vi "stepper graphics controller -- V3.vi"(6 "stepper motor state":T2, 7 "slider setter action":T3, 8 "stepper graphics internal state":T1, 10 "value":dbl=1.0 format="%#_13g") -> (0 "stepper graphics internal state OUT":T1)   [LabVIEW 2018]
uses:
  slider setter action.ctl
  stepper motor state.ctl
  stepper graphics internal state.ctl
  2Dwindow.ctl
  slider action.ctl
  cursor action.ctl
  generate linear region.vi
  generate linear region --complex -- win cen.vi
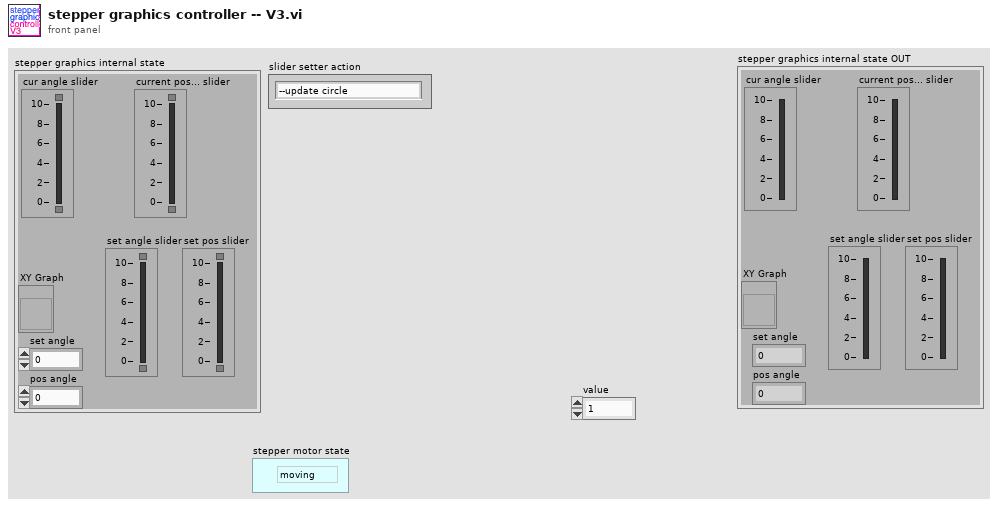
[diagram p1: front panel]
types:
  T1 = typedef "stepper graphics internal state.ctl" = cluster{"set pos slider":refnum<vi>, "cur angle slider":refnum<vi>, "XY Graph":refnum<vi>, "set angle":dbl, "pos angle":dbl, "set angle slider":refnum<vi>, "current pos... slider":refnum<vi>}
  T2 = typedef "stepper motor state.ctl" = enum16{"moving", "stopped"}
  T3 = typedef "slider setter action.ctl" = enum16{"--update circle", "set step slider moves", "cursor moves", "current pos changed", "init", "void", "--draw current lie", "--draw set line", "--move current step slider", "--move set step slider", "--draw limit lines", "check", "--move set angle slider", "--move current angle slider", "set angle slider moves", "--move cursor", "set set step", "set current step"}
  T4 = typedef "2Dwindow.ctl" = cluster{"window y":dbl, "center x":dbl, "center y":dbl, "window x":dbl}
  T5 = typedef "slider action.ctl" = enum16{"check", "copy range", "set from value", "set from ratio", "set from slider", "read using other slider"}
  T6 = typedef "cursor action.ctl" = enum16{"range", "read", "write", "check", "zoom out", "smart zoom out", "zoom to aspect ratio 1", "zoom to win", "zoom out 20%", "zoom in 20%", "-empty", "smart zoom out&aspect", "move range left 20%", "move range right 20%", "move range up 20%", "move range down 20%", "zoom to X win", "zoom to Y win", "zoom out X", "zoom out Y", "zoom in X", "zoom in Y", "check plot scale"}
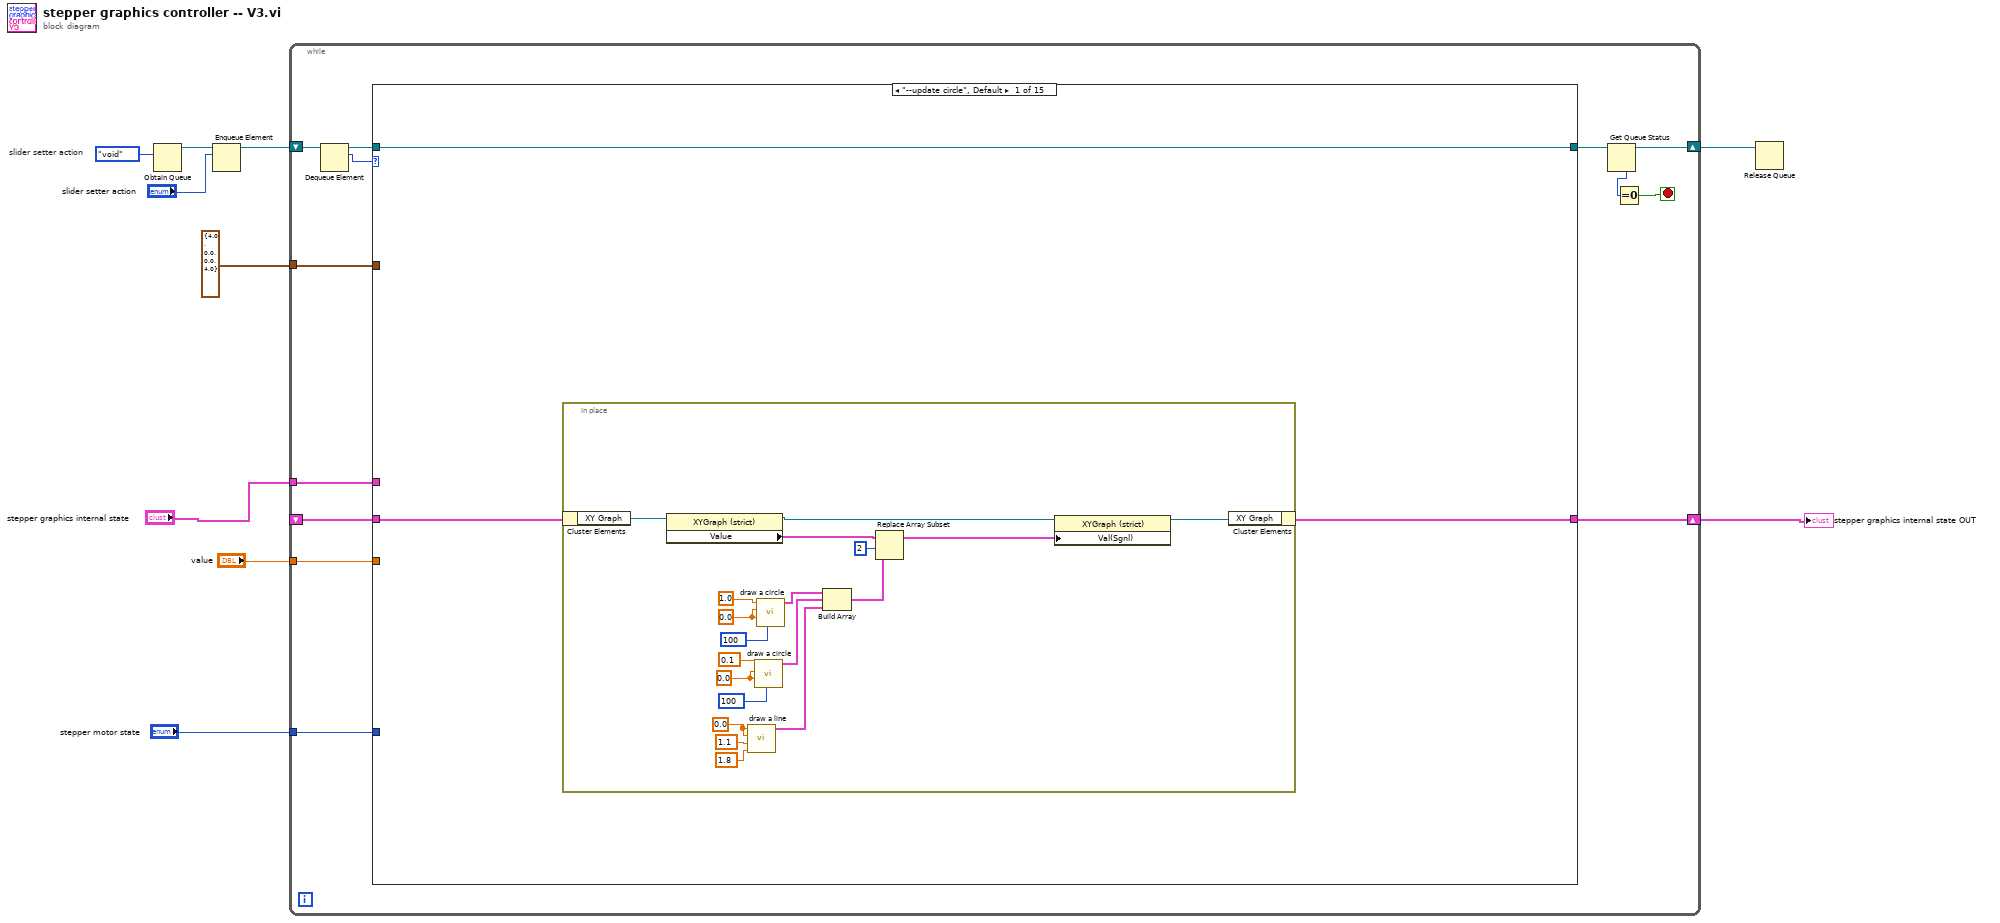
[diagram p0: block diagram]
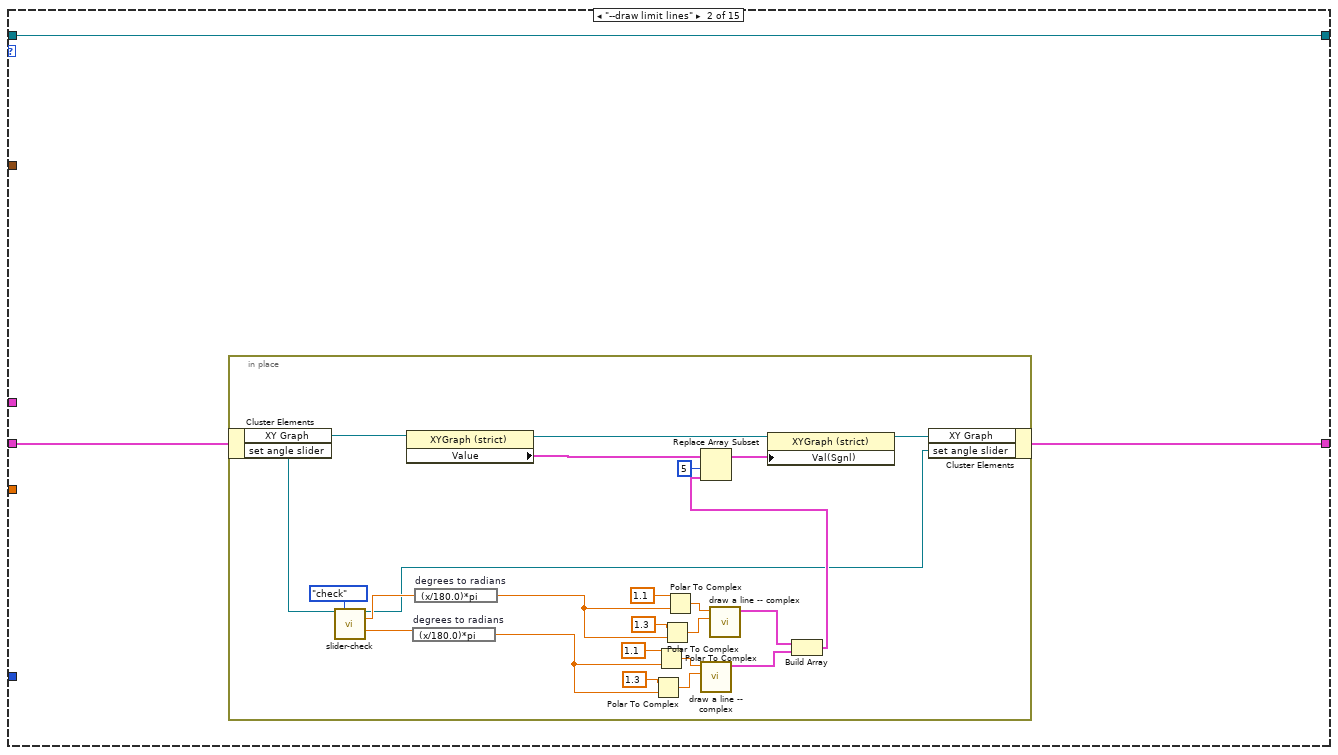
[diagram p2: hidden frame]
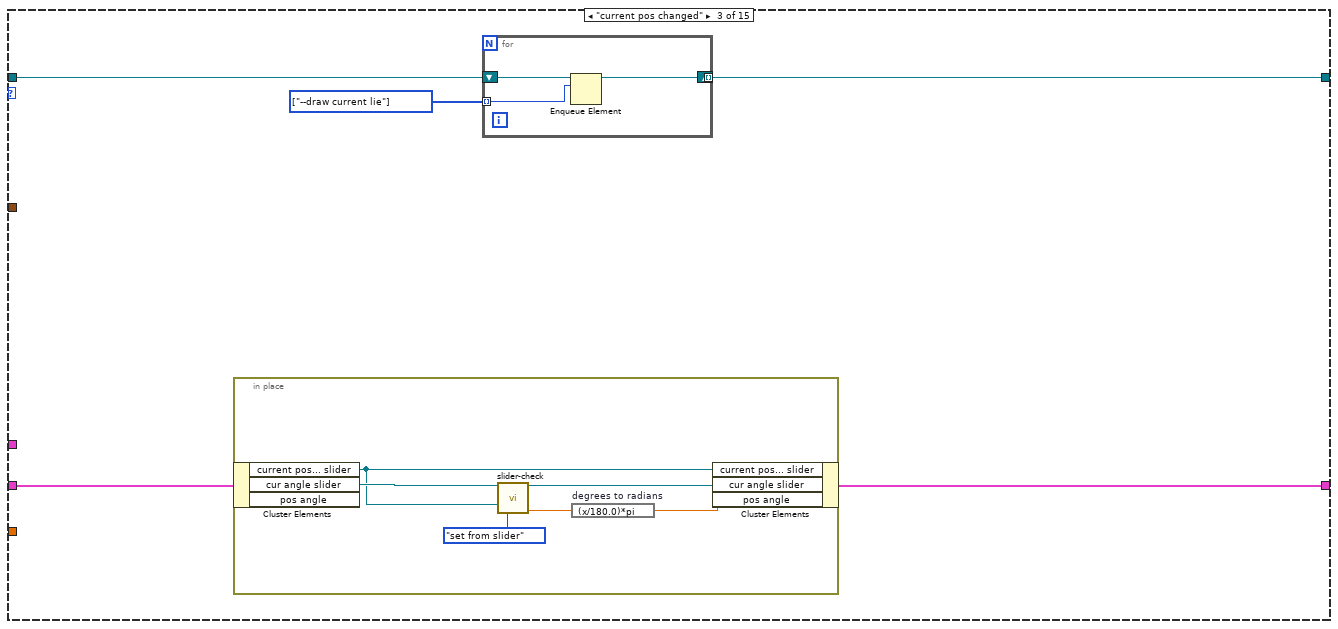
[diagram p3: hidden frame]
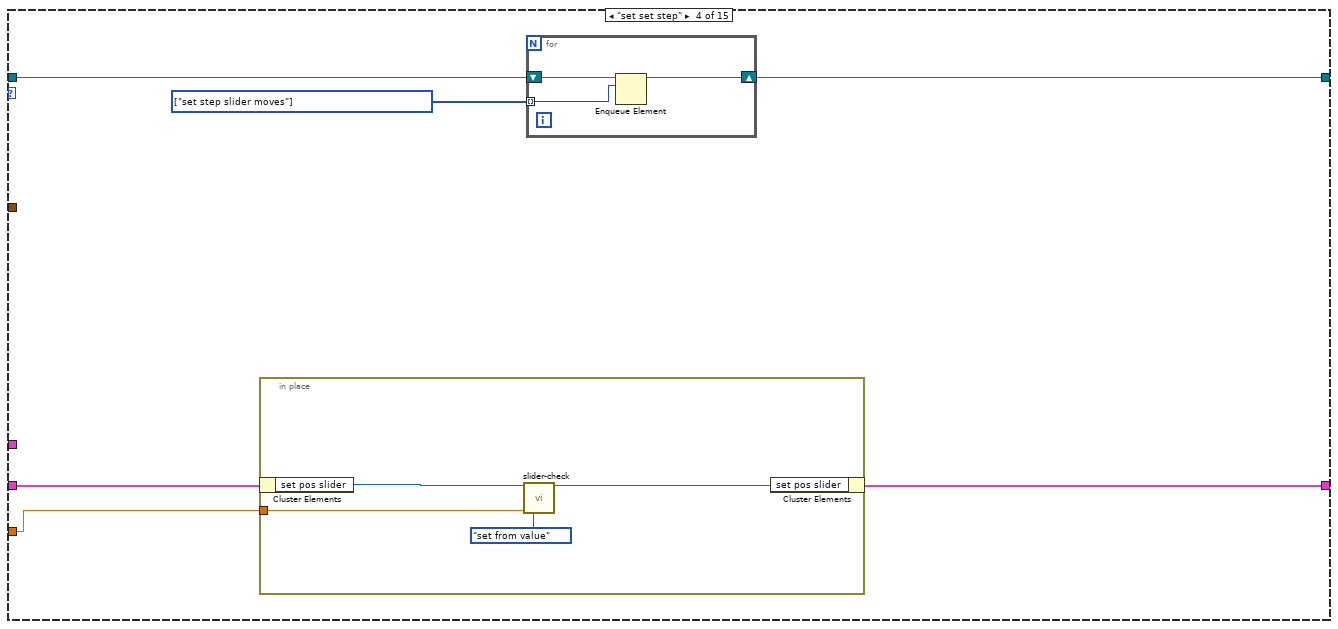
[diagram p4: hidden frame]
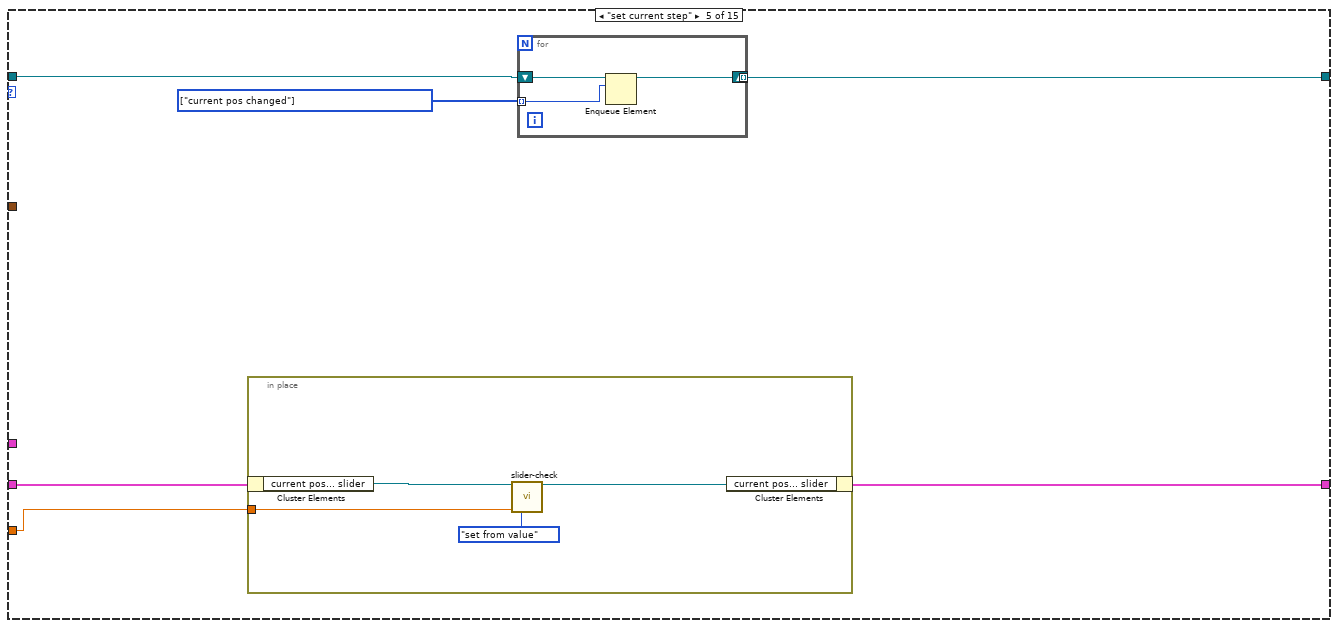
[diagram p5: hidden frame]
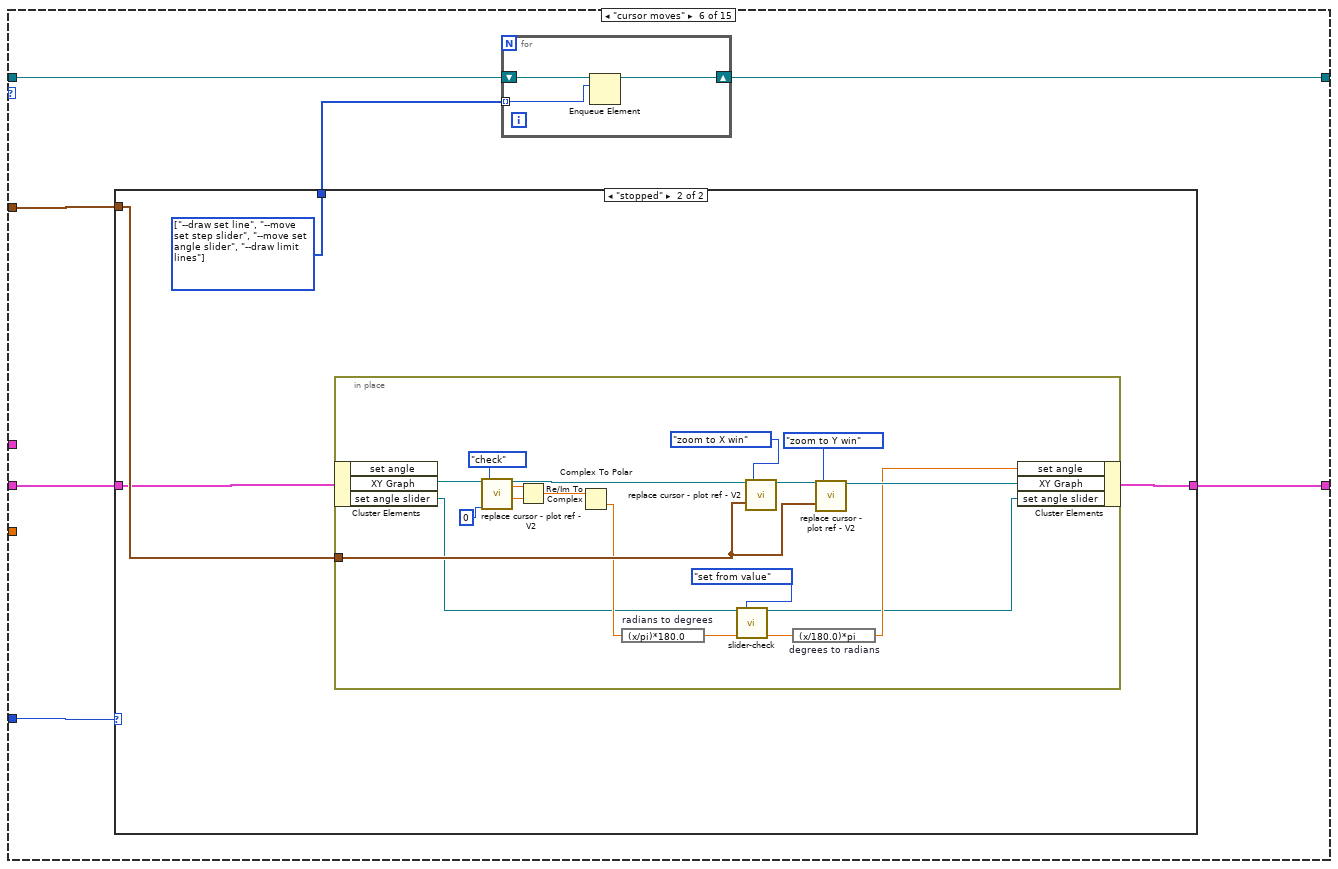
[diagram p6: hidden frame]
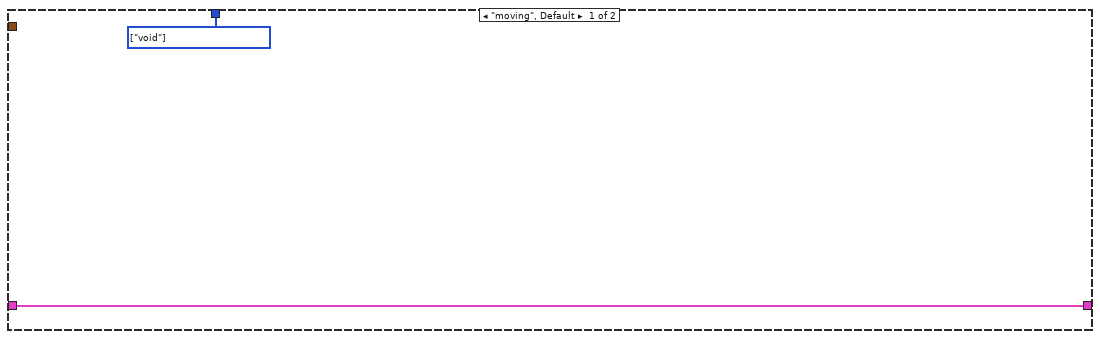
[diagram p7: hidden frame]
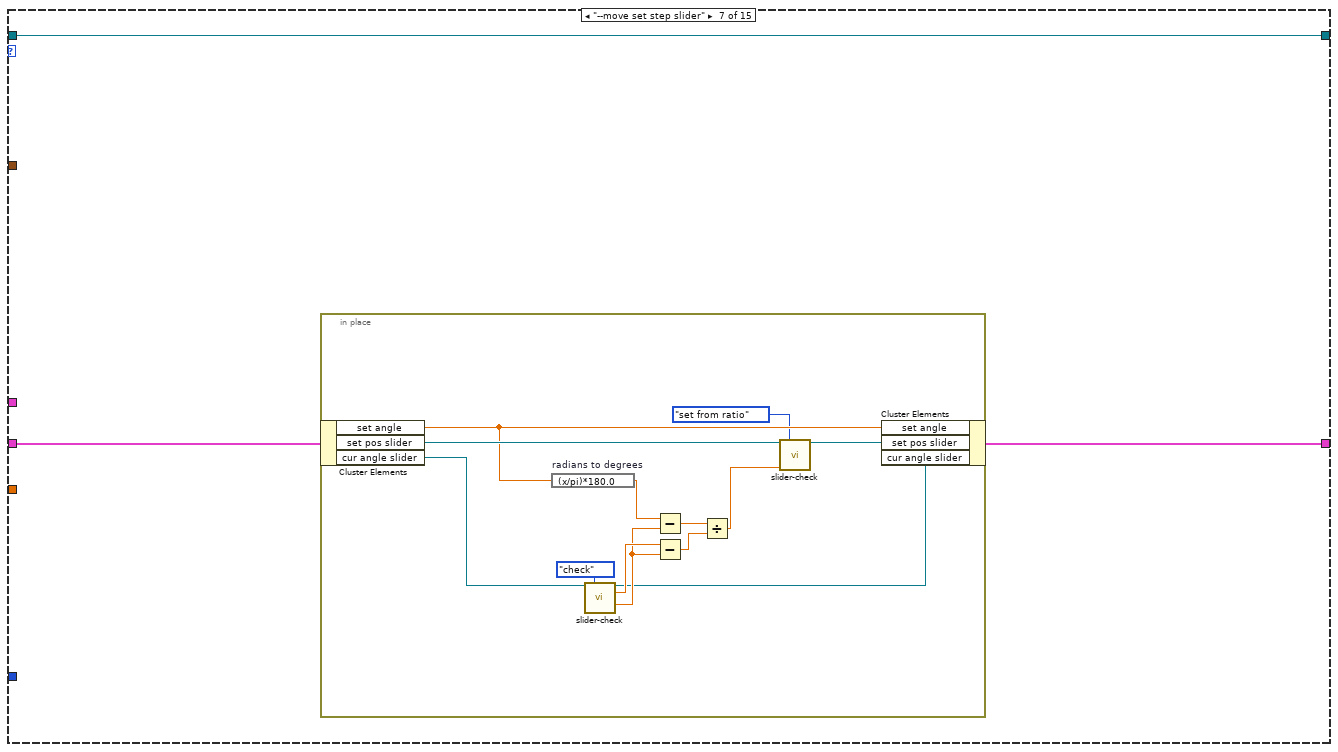
[diagram p8: hidden frame]
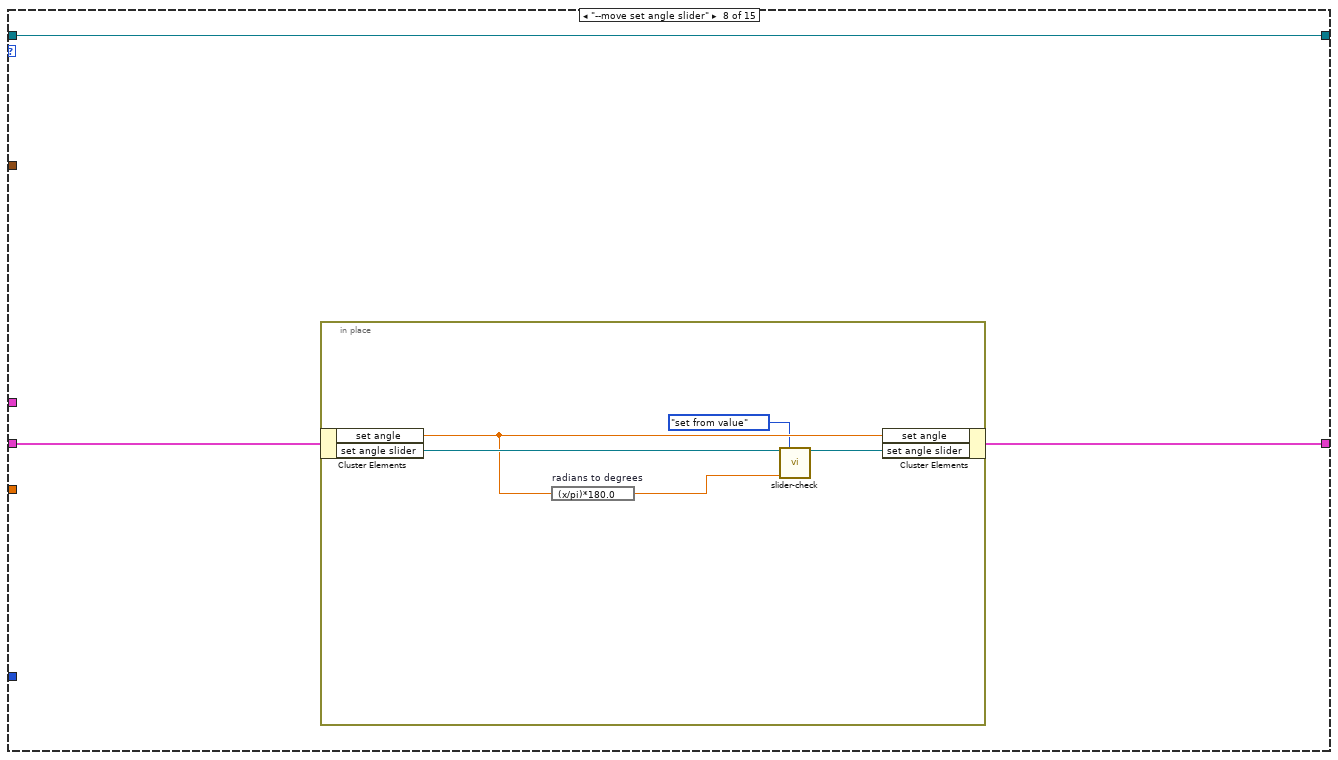
[diagram p9: hidden frame]
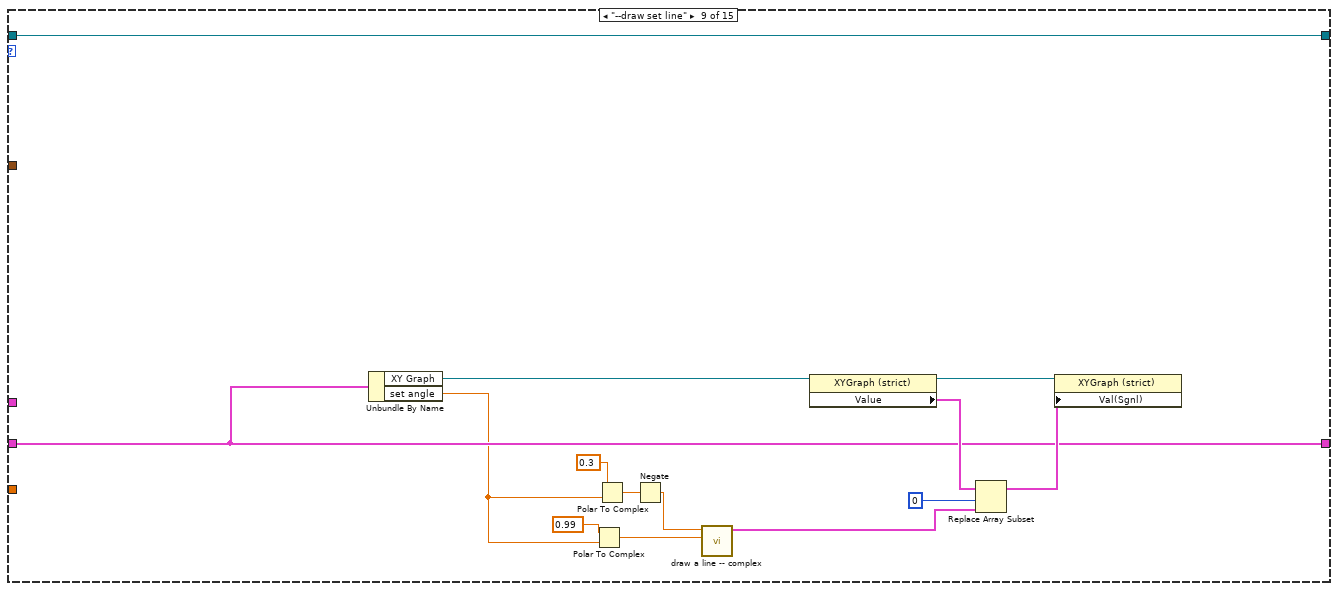
[diagram p10: hidden frame]
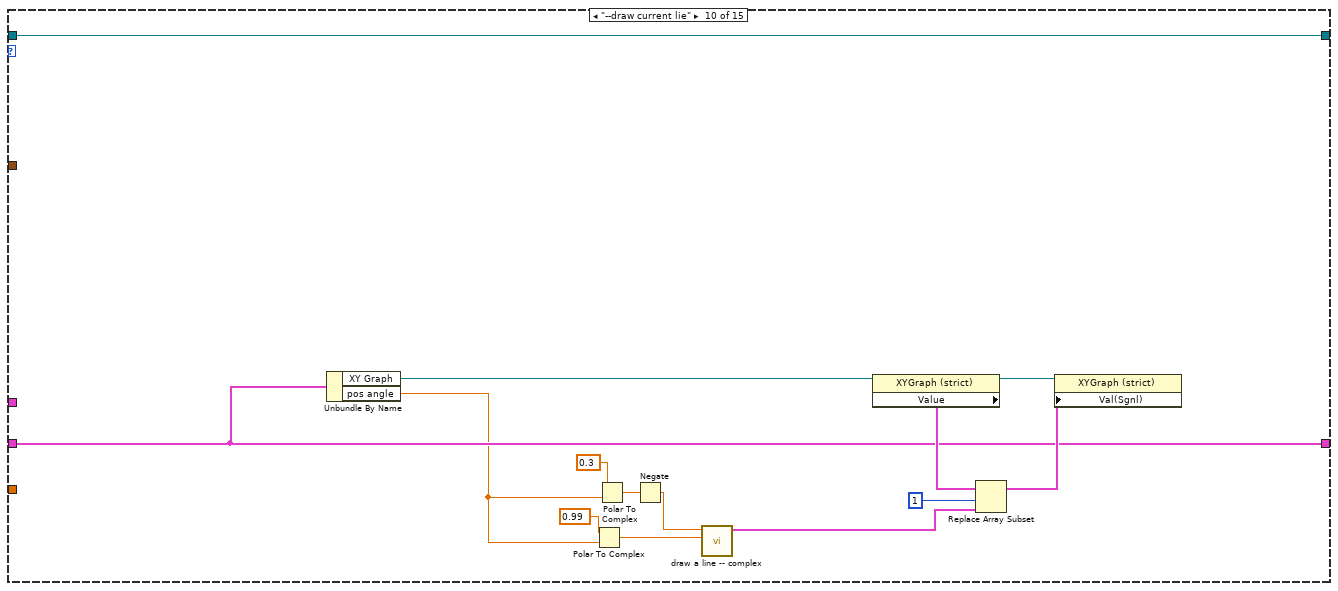
[diagram p11: hidden frame]
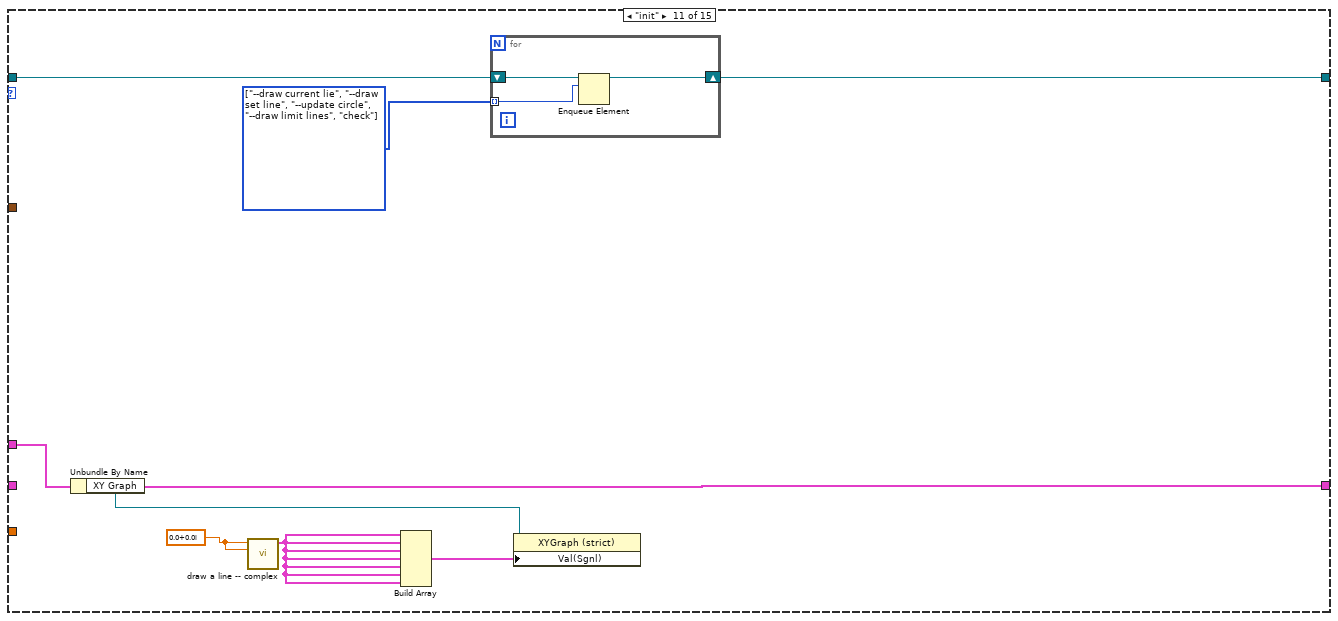
[diagram p12: hidden frame]
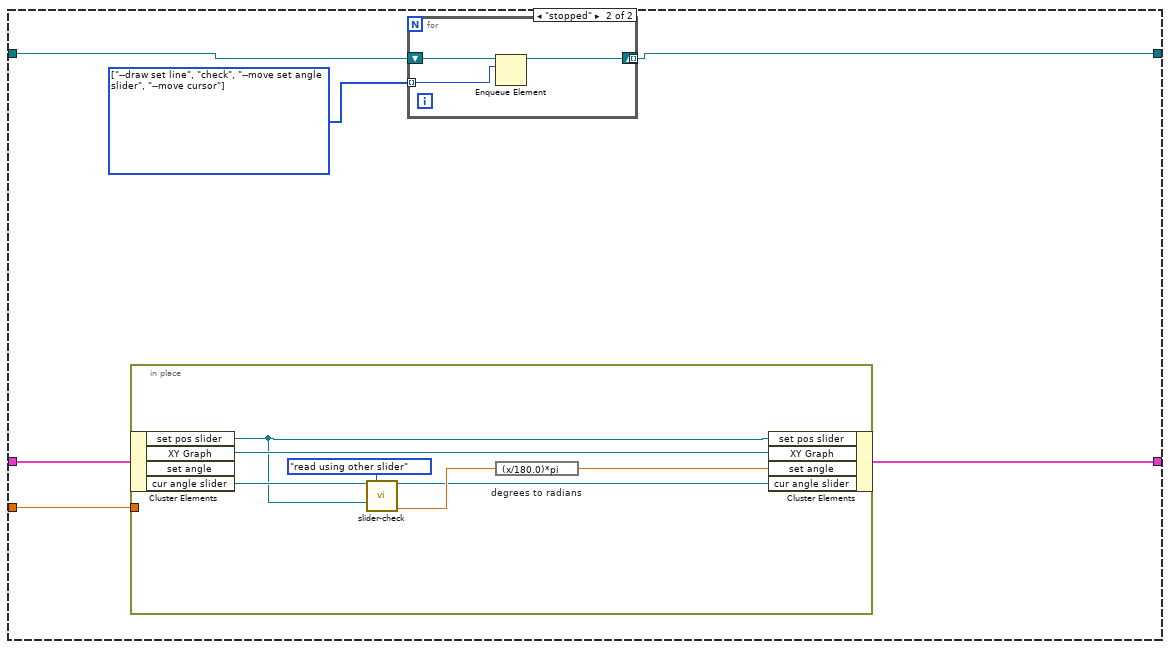
[diagram p14: hidden frame]
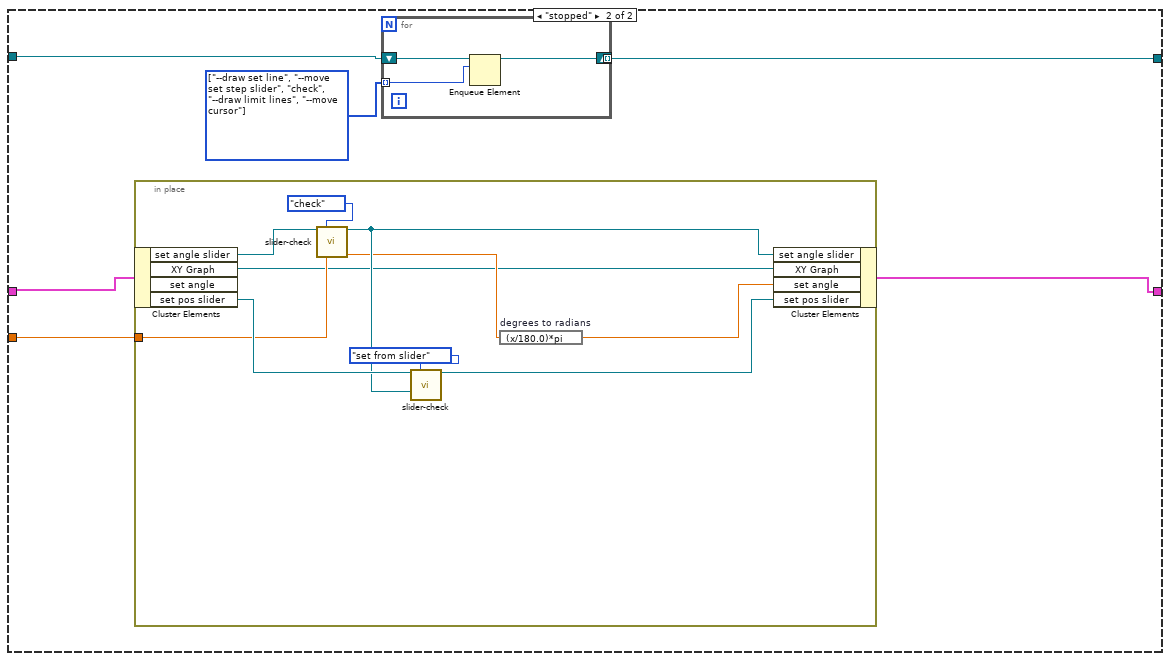
[diagram p16: hidden frame]
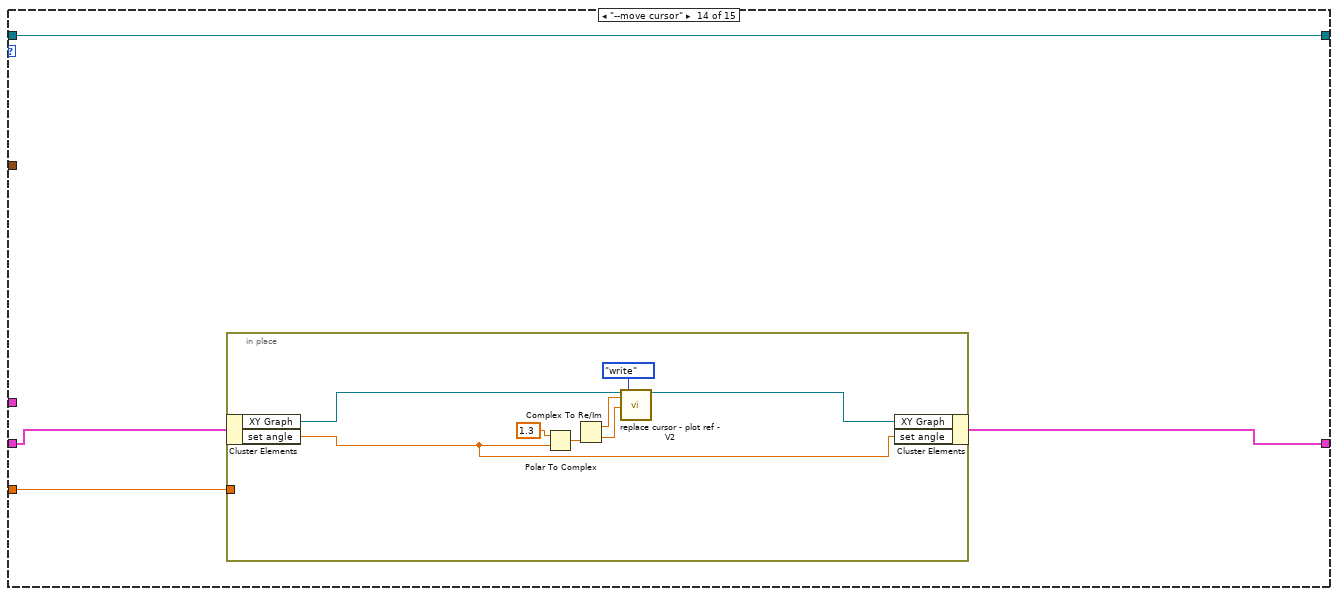
[diagram p17: hidden frame]
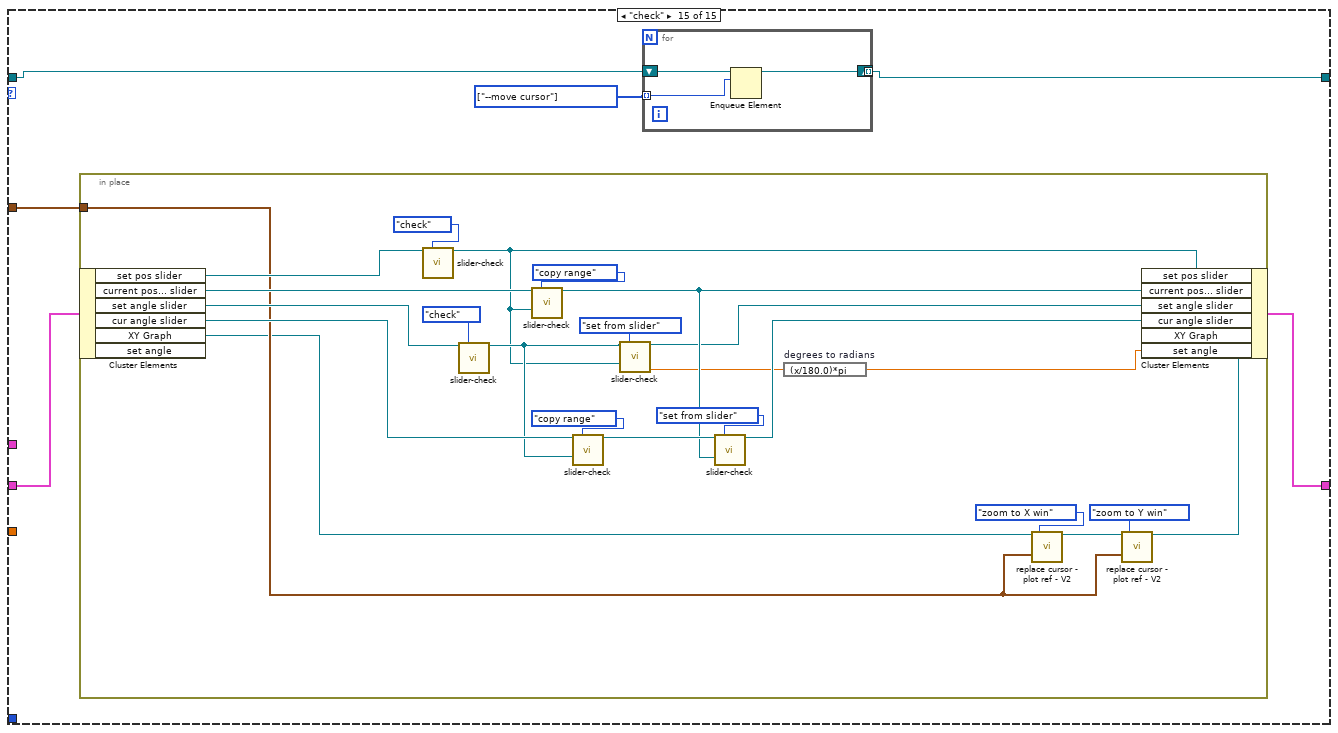
[diagram p18: hidden frame]
diagram:
  w7 = slider_setter_action."void"  # slider setter action
  n1 = Obtain Queue(element data type=w7) -> (queue out=w6:refnum<queue>)  [unwired: 4 in, 2 out]
  n2 = Enqueue Element(queue=w6, element="slider setter action") -> (queue out=w5:refnum<queue>)  [unwired: 2 in, 2 out]
  n3 = while {
    tunnel: "stepper motor state" -> [w23]
    tunnel: T4 {"window y"=4.0, "center x"=0.0, "center y"=0.0, "window x"=4.0} ("window IN") -> [w22]
    shift-right: [w15] -> w3
    shift-left: w5 -> [w17]
    tunnel: "stepper graphics internal state" -> [w21]
    shift-right: [w20] -> w1
    shift-left: _ -> [w19]
    tunnel: "value" -> [w18]
    stop <- w11 stop-if-true
    n4 = Dequeue Element(queue=w17) -> (queue out=w14:refnum<queue>, element=w16:T3)  [unwired: 2 in, 2 out]
    n5 = case shown="\"--update circle\", Default" w16 {
      tunnel: w23 -> [_ _ _ _ _ w119 _ _ _ _ _ w216 w240 _ _]
      tunnel: w22 -> [_ _ _ _ _ w118 _ _ _ _ _ _ _ _ w277]
      tunnel: w21 -> [_ _ _ _ _ _ _ _ _ _ w204 _ _ _ _]
      tunnel: [w25 w47 w76 w91 w104 w117 w149 w165 w175 w189 w204 w215 w239 w265 w279] -> w20
      tunnel: w19 -> [w26 w48 w77 w92 w105 w116 w150 w166 w175 w189 _ w214 w238 w264 w278]
      tunnel: w18 -> [_ _ _ w90 w103 _ _ _ _ _ _ w213 w237 w263 _]
      tunnel: w14 -> [w24 w46 w74 w88 w101 w114 w148 w164 w172 w186 w201 w212 w236 w262 w275]
      tunnel: [w24 w46 w73 w87 w100 w113 w148 w164 w172 w186 w200 w211 w235 w262 w274] -> w13
      frame "--update circle", Default {
        n6 = in-place {
          w39 = 0.0 ("center x")
          w42 = 0.0 ("x0")
          w45 = 0.0 ("center x")
          n7 = in-place-cluster #1(w26) -> ("XY Graph"=w35:refnum<vi>)
          n8 = property class="XYGraph (strict)"(reference=w35) -> (reference out=w34:refnum<vi>, "Value"=w33:cluster{dbl[], dbl[]}[])  [unwired: 1 in, 1 out]
          n9 = call "draw a line.vi"("y1"=1.8 ("x0"), "y0"=1.1 ("x0"), "x1"=w42, "x0"=w42) -> ("output cluster"=w29:cluster{dbl[], dbl[]})  [unwired: 7 in]
          n10 = call "draw a circle.vi"("number of points"=100, "center Y"=w39, "center x"=w39, "radius"=0.1) -> ("output cluster"=w30:cluster{dbl[], dbl[]})  [unwired: 7 in]
          n11 = call "draw a circle.vi"("number of points"=100, "center Y"=w45, "center x"=w45, "radius"=1.0) -> ("output cluster"=w31:cluster{dbl[], dbl[]})  [unwired: 7 in]
          n12 = Build Array(w31, w30, w29) -> (w28:cluster{dbl[], dbl[]}[])
          n13 = Replace Array Subset(array=w33, new element=w28, index=2) -> (w27:cluster{dbl[], dbl[]}[])
          n14 = property class="XYGraph (strict)"(reference=w34, "Val(Sgnl)"=w27) -> (reference out=w36:refnum<vi>)  [unwired: 1 in, 1 out]
          n15 = in-place-cluster #1("XY Graph"=w36) -> (w25:T1)
        }
      }
      frame "--draw limit lines" {
        n16 = in-place {
          n17 = in-place-cluster #2(w48) -> ("XY Graph"=w71:refnum<vi>, "set angle slider"=w65:refnum<vi>)
          n18 = call "slider-check.vi"("slider in"=w65, "slider action"=slider_action."check") -> ("slider out"=w49:refnum<vi>, "max"=w64:dbl, "min"=w63:dbl)  [unwired: 9 in, 2 out]
          n19 = property class="XYGraph (strict)"(reference=w71) -> (reference out=w70:refnum<vi>, "Value"=w69:cluster{dbl[], dbl[]}[])  [unwired: 1 in, 1 out]
          n20 = expression code="(x/180.0)*pi" "degrees to radians"(w63) -> (w53:dbl)
          n21 = expression code="(x/180.0)*pi" "degrees to radians"(w64) -> (w59:dbl)
          n22 = Polar To Complex(1:w53, 2:1.3 ("x")) -> (0:w55:cdb)
          n23 = Polar To Complex(1:w53, 2:1.1 ("x")) -> (0:w54:cdb)
          n24 = Polar To Complex(1:w59, 2:1.3 ("x")) -> (0:w60:cdb)
          n25 = Polar To Complex(1:w59, 2:1.1 ("x")) -> (0:w58:cdb)
          n26 = call "draw a line -- complex.vi"("x1"=w55, "x0"=w54) -> ("output cluster"=w51:cluster{dbl[], dbl[]})  [unwired: 9 in]
          n27 = call "draw a line -- complex.vi"("x1"=w60, "x0"=w58) -> ("output cluster"=w52:cluster{dbl[], dbl[]})  [unwired: 9 in]
          n28 = Build Array(w52, w51) -> (w50:cluster{dbl[], dbl[]}[])
          n29 = Replace Array Subset(array=w69, new element=w50, index=5) -> (w67:cluster{dbl[], dbl[]}[])
          n30 = property class="XYGraph (strict)"(reference=w70, "Val(Sgnl)"=w67) -> (reference out=w72:refnum<vi>)  [unwired: 1 in, 1 out]
          n31 = in-place-cluster #2("XY Graph"=w72, "set angle slider"=w49) -> (w47:T1)
        }
      }
      frame "current pos changed" {
        w75 = T3[] [enum."--draw current lie"] items=["--update circle", "set step slider moves", "cursor moves", "current pos changed", "init", "void", "--draw current lie", "--draw set line", "--move current step slider", "--move set step slider", "--draw limit lines", "check", "--move set angle slider", "--move current angle slider", "set angle slider moves", "--move cursor", "set set step", "set current step"] ("action list IN")
        n32 = in-place {
          n33 = in-place-cluster #3(w77) -> ("current pos... slider"=w81:refnum<vi>, "cur angle slider"=w86:refnum<vi>)  [unwired: 1 out]
          n34 = call "slider-check.vi"("slider in"=w86, "slider action"=slider_action."set from slider", "slider from"=w81) -> ("slider out"=w83:refnum<vi>, "value OUT"=w85:dbl)  [unwired: 8 in, 3 out]
          n35 = expression code="(x/180.0)*pi" "degrees to radians"(w85) -> (w84:dbl)
          n36 = in-place-cluster #3("current pos... slider"=w81, "cur angle slider"=w83, "pos angle"=w84) -> (w76:T1)
        }
        n37 = for {
          shift-right: [w78] -> w73
          shift-left: w74 -> [w80]
          tunnel: w75 -> [w79] mode=indexing
          tunnel: [w78] -> _ mode=indexing
          n38 = Enqueue Element(queue=w80, element=w79) -> (queue out=w78:refnum<queue>)  [unwired: 2 in, 2 out]
        }
      }
      frame "set set step" {
        w89 = T3[] [enum."set step slider moves"] items=["--update circle", "set step slider moves", "cursor moves", "current pos changed", "init", "void", "--draw current lie", "--draw set line", "--move current step slider", "--move set step slider", "--draw limit lines", "check", "--move set angle slider", "--move current angle slider", "set angle slider moves", "--move cursor", "set set step", "set current step"] ("action list IN")
        n39 = in-place {
          in-place-border: w90 -> [w96]
          n40 = in-place-cluster #4(w92) -> ("set pos slider"=w99:refnum<vi>)
          n41 = call "slider-check.vi"("slider in"=w99, "slider action"=slider_action."set from value", "value IN"=w96) -> ("slider out"=w98:refnum<vi>)  [unwired: 8 in, 4 out]
          n42 = in-place-cluster #4("set pos slider"=w98) -> (w91:T1)
        }
        n43 = for {
          shift-right: [w93] -> w87
          shift-left: w88 -> [w95]
          tunnel: w89 -> [w94] mode=indexing
          n44 = Enqueue Element(queue=w95, element=w94) -> (queue out=w93:refnum<queue>)  [unwired: 2 in, 2 out]
        }
      }
      frame "set current step" {
        w102 = T3[] [enum."current pos changed"] items=["--update circle", "set step slider moves", "cursor moves", "current pos changed", "init", "void", "--draw current lie", "--draw set line", "--move current step slider", "--move set step slider", "--draw limit lines", "check", "--move set angle slider", "--move current angle slider", "set angle slider moves", "--move cursor", "set set step", "set current step"] ("action list IN")
        n45 = in-place {
          in-place-border: w103 -> [w109]
          n46 = in-place-cluster #5(w105) -> ("current pos... slider"=w112:refnum<vi>)
          n47 = call "slider-check.vi"("slider in"=w112, "slider action"=slider_action."set from value", "value IN"=w109) -> ("slider out"=w111:refnum<vi>)  [unwired: 8 in, 4 out]
          n48 = in-place-cluster #5("current pos... slider"=w111) -> (w104:T1)
        }
        n49 = for {
          shift-right: [w106] -> w100
          shift-left: w101 -> [w108]
          tunnel: w102 -> [w107] mode=indexing
          tunnel: [w106] -> _ mode=indexing
          n50 = Enqueue Element(queue=w108, element=w107) -> (queue out=w106:refnum<queue>)  [unwired: 2 in, 2 out]
        }
      }
      frame "cursor moves" {
        n51 = case shown="\"stopped\"" w119 {
          tunnel: w118 -> [_ w128]
          tunnel: [w124 w127] -> w117
          tunnel: w116 -> [w124 w126]
          tunnel: [w123 w125] -> w115
          frame "moving", Default {
            w123 = T3[] [enum."void"] items=["--update circle", "set step slider moves", "cursor moves", "current pos changed", "init", "void", "--draw current lie", "--draw set line", "--move current step slider", "--move set step slider", "--draw limit lines", "check", "--move set angle slider", "--move current angle slider", "set angle slider moves", "--move cursor", "set set step", "set current step"] ("action list IN")
          }
          frame "stopped" {
            w125 = T3[] [enum."--draw set line", enum."--move set step slider", enum."--move set angle slider", enum."--draw limit lines"] items=["--update circle", "set step slider moves", "cursor moves", "current pos changed", "init", "void", "--draw current lie", "--draw set line", "--move current step slider", "--move set step slider", "--draw limit lines", "check", "--move set angle slider", "--move current angle slider", "set angle slider moves", "--move cursor", "set set step", "set current step"] ("action list IN")
            n52 = in-place {
              in-place-border: w128 -> [w140]
              n53 = in-place-cluster #6(w126) -> ("XY Graph"=w138:refnum<vi>, "set angle slider"=w134:refnum<vi>)  [unwired: 1 out]
              n54 = call "replace cursor - plot ref - V2.vi"("Plot ref in"=w138, "cursor index"=0, "cursor action"=cursor_action."check") -> ("Plot ref out"=w139:refnum<vi>, "read X"=w145:dbl, "read Y"=w144:dbl)  [unwired: 13 in, 1 out]
              n55 = Re/Im To Complex(1:w144, 2:w145) -> (0:w143:cdb)
              n56 = Complex To Polar(r * e^(i*theta)=w143) -> (theta=w135:dbl)  [unwired: 1 out]
              n57 = expression code="(x/pi)*180.0" "radians to degrees"(w135) -> (w133:dbl)
              n58 = call "slider-check.vi"("slider in"=w134, "slider action"=slider_action."set from value", "value IN"=w133) -> ("slider out"=w129:refnum<vi>, "value OUT"=w131:dbl)  [unwired: 8 in, 3 out]
              n59 = call "replace cursor - plot ref - V2.vi"("Plot ref in"=w139, "window IN"=w140, "cursor action"=cursor_action."zoom to X win") -> ("Plot ref out"=w137:refnum<vi>)  [unwired: 13 in, 3 out]
              n60 = expression code="(x/180.0)*pi" "degrees to radians"(w131) -> (w130:dbl)
              n61 = call "replace cursor - plot ref - V2.vi"("Plot ref in"=w137, "window IN"=w140, "cursor action"=cursor_action."zoom to Y win") -> ("Plot ref out"=w136:refnum<vi>)  [unwired: 13 in, 3 out]
              n62 = in-place-cluster #6("set angle"=w130, "XY Graph"=w136, "set angle slider"=w129) -> (w127:T1)
            }
          }
        }
        n63 = for {
          shift-right: [w121] -> w113
          shift-left: w114 -> [w122]
          tunnel: w115 -> [w120] mode=indexing
          n64 = Enqueue Element(queue=w122, element=w120) -> (queue out=w121:refnum<queue>)  [unwired: 2 in, 2 out]
        }
      }
      frame "--move set step slider" {
        n65 = in-place {
          n66 = in-place-cluster #7(w150) -> ("set angle"=w153:dbl, "set pos slider"=w155:refnum<vi>, "cur angle slider"=w156:refnum<vi>)
          n67 = expression code="(x/pi)*180.0" "radians to degrees"(w153) -> (w157:dbl)
          n68 = call "slider-check.vi"("slider in"=w156, "slider action"=slider_action."check") -> ("slider out"=w152:refnum<vi>, "max"=w162:dbl, "min"=w161:dbl)  [unwired: 9 in, 2 out]
          n69 = Subtract(x=w157, y=w161) -> (x-y=w160:dbl)
          n70 = Subtract(x=w162, y=w161) -> (x-y=w159:dbl)
          n71 = Divide(x=w160, y=w159) -> (x/y=w158:dbl)
          n72 = call "slider-check.vi"("slider in"=w155, "slider action"=slider_action."set from ratio", "value IN"=w158) -> ("slider out"=w154:refnum<vi>)  [unwired: 8 in, 4 out]
          n73 = in-place-cluster #7("set angle"=w153, "set pos slider"=w154, "cur angle slider"=w152) -> (w149:T1)
        }
      }
      frame "--move set angle slider" {
        n74 = in-place {
          n75 = in-place-cluster #8(w166) -> ("set angle"=w169:dbl, "set angle slider"=w171:refnum<vi>)
          n76 = expression code="(x/pi)*180.0" "radians to degrees"(w169) -> (w168:dbl)
          n77 = call "slider-check.vi"("slider in"=w171, "slider action"=slider_action."set from value", "value IN"=w168) -> ("slider out"=w170:refnum<vi>)  [unwired: 8 in, 4 out]
          n78 = in-place-cluster #8("set angle"=w169, "set angle slider"=w170) -> (w165:T1)
        }
      }
      frame "--draw set line" {
        n79 = Unbundle By Name(w175) -> ("XY Graph"=w173:refnum<vi>, "set angle"=w174:dbl)
        n80 = Polar To Complex(1:w174, 2:0.99 ("x")) -> (0:w177:cdb)
        n81 = Polar To Complex(1:w174, 2:0.3 ("x")) -> (0:w179:cdb)
        n82 = Negate(x=w179) -> (-x=w178:cdb)
        n83 = call "draw a line -- complex.vi"("x1"=w177, "x0"=w178) -> ("output cluster"=w176:cluster{dbl[], dbl[]})  [unwired: 9 in]
        n84 = property class="XYGraph (strict)"(reference=w173) -> (reference out=w185:refnum<vi>, "Value"=w184:cluster{dbl[], dbl[]}[])  [unwired: 1 in, 1 out]
        n85 = Replace Array Subset(array=w184, new element=w176, index=0) -> (w183:cluster{dbl[], dbl[]}[])
        n86 = property class="XYGraph (strict)"(reference=w185, "Val(Sgnl)"=w183) -> ()  [unwired: 1 in, 2 out]
      }
      frame "--draw current lie" {
        n87 = Unbundle By Name(w189) -> ("XY Graph"=w187:refnum<vi>, "pos angle"=w188:dbl)
        n88 = Polar To Complex(1:w188, 2:0.99 ("x")) -> (0:w191:cdb)
        n89 = Polar To Complex(1:w188, 2:0.3 ("x")) -> (0:w193:cdb)
        n90 = Negate(x=w193) -> (-x=w192:cdb)
        n91 = call "draw a line -- complex.vi"("x1"=w191, "x0"=w192) -> ("output cluster"=w190:cluster{dbl[], dbl[]})  [unwired: 9 in]
        n92 = property class="XYGraph (strict)"(reference=w187) -> (reference out=w199:refnum<vi>, "Value"=w198:cluster{dbl[], dbl[]}[])  [unwired: 1 in, 1 out]
        n93 = Replace Array Subset(array=w198, new element=w190, index=1) -> (w197:cluster{dbl[], dbl[]}[])
        n94 = property class="XYGraph (strict)"(reference=w199, "Val(Sgnl)"=w197) -> ()  [unwired: 1 in, 2 out]
      }
      frame "init" {
        w206 = cdb 0.0+0.0i ("x0")
        w202 = T3[] [enum."--draw current lie", enum."--draw set line", enum."--update circle", enum."--draw limit lines", enum."check"] items=["--update circle", "set step slider moves", "cursor moves", "current pos changed", "init", "void", "--draw current lie", "--draw set line", "--move current step slider", "--move set step slider", "--draw limit lines", "check", "--move set angle slider", "--move current angle slider", "set angle slider moves", "--move cursor", "set set step", "set current step"] ("action list IN")
        n95 = Unbundle By Name(w204) -> ("XY Graph"=w203:refnum<vi>)
        n96 = call "draw a line -- complex.vi"("x1"=w206, "x0"=w206) -> ("output cluster"=w205:cluster{dbl[], dbl[]})  [unwired: 9 in]
        n97 = Build Array(w205, w205, w205, w205, w205, w205, w205) -> (w207:cluster{dbl[], dbl[]}[])
        n98 = for {
          shift-right: [w208] -> w200
          shift-left: w201 -> [w210]
          tunnel: w202 -> [w209] mode=indexing
          n99 = Enqueue Element(queue=w210, element=w209) -> (queue out=w208:refnum<queue>)  [unwired: 2 in, 2 out]
        }
        n100 = property class="XYGraph (strict)"(reference=w203, "Val(Sgnl)"=w207) -> ()  [unwired: 1 in, 2 out]
      }
      frame "set step slider moves" {
        n101 = case shown="\"moving\", Default" w216 {
          tunnel: w214 -> [w218 w224]
          tunnel: [w218 w223] -> w215
          tunnel: w213 -> [_ w222]
          tunnel: w212 -> [w217 w220]
          tunnel: [w217 w219] -> w211
          frame "moving", Default {
          }
          frame "stopped" {
            w221 = T3[] [enum."--draw set line", enum."check", enum."--move set angle slider", enum."--move cursor"] items=["--update circle", "set step slider moves", "cursor moves", "current pos changed", "init", "void", "--draw current lie", "--draw set line", "--move current step slider", "--move set step slider", "--draw limit lines", "check", "--move set angle slider", "--move current angle slider", "set angle slider moves", "--move cursor", "set set step", "set current step"] ("action list IN")
            n102 = in-place {
              in-place-border: w222 -> [_]
              n103 = in-place-cluster #9(w224) -> ("set pos slider"=w230:refnum<vi>, "XY Graph"=w231:refnum<vi>, "cur angle slider"=w233:refnum<vi>)  [unwired: 1 out]
              n104 = call "slider-check.vi"("slider in"=w233, "slider action"=slider_action."read using other slider", "slider from"=w230) -> ("slider out"=w228:refnum<vi>, "value OUT"=w229:dbl)  [unwired: 8 in, 3 out]
              n105 = expression code="(x/180.0)*pi" "degrees to radians"(w229) -> (w232:dbl)
              n106 = in-place-cluster #9("set pos slider"=w230, "XY Graph"=w231, "set angle"=w232, "cur angle slider"=w228) -> (w223:T1)
            }
            n107 = for {
              shift-right: [w225] -> w219
              shift-left: w220 -> [w227]
              tunnel: w221 -> [w226] mode=indexing
              tunnel: [w225] -> _ mode=indexing
              n108 = Enqueue Element(queue=w227, element=w226) -> (queue out=w225:refnum<queue>)  [unwired: 2 in, 2 out]
            }
          }
        }
      }
      frame "set angle slider moves" {
        n109 = case shown="\"moving\", Default" w240 {
          tunnel: w238 -> [w242 w248]
          tunnel: [w242 w247] -> w239
          tunnel: w237 -> [_ w246]
          tunnel: w236 -> [w241 w244]
          tunnel: [w241 w243] -> w235
          frame "moving", Default {
          }
          frame "stopped" {
            w245 = T3[] [enum."--draw set line", enum."--move set step slider", enum."check", enum."--draw limit lines", enum."--move cursor"] items=["--update circle", "set step slider moves", "cursor moves", "current pos changed", "init", "void", "--draw current lie", "--draw set line", "--move current step slider", "--move set step slider", "--draw limit lines", "check", "--move set angle slider", "--move current angle slider", "set angle slider moves", "--move cursor", "set set step", "set current step"] ("action list IN")
            n110 = in-place {
              in-place-border: w246 -> [w256]
              n111 = in-place-cluster #10(w248) -> ("set angle slider"=w259:refnum<vi>, "XY Graph"=w252:refnum<vi>, "set pos slider"=w258:refnum<vi>)  [unwired: 1 out]
              n112 = call "slider-check.vi"("slider in"=w259, "slider action"=slider_action."check", "default"=w256) -> ("slider out"=w255:refnum<vi>, "value OUT"=w253:dbl)  [unwired: 8 in, 3 out]
              n113 = call "slider-check.vi"("slider in"=w258, "slider action"=slider_action."set from slider", "slider from"=w255) -> ("slider out"=w254:refnum<vi>)  [unwired: 8 in, 4 out]
              n114 = expression code="(x/180.0)*pi" "degrees to radians"(w253) -> (w257:dbl)
              n115 = in-place-cluster #10("set angle slider"=w255, "XY Graph"=w252, "set angle"=w257, "set pos slider"=w254) -> (w247:T1)
            }
            n116 = for {
              shift-right: [w249] -> w243
              shift-left: w244 -> [w251]
              tunnel: w245 -> [w250] mode=indexing
              tunnel: [w249] -> _ mode=indexing
              n117 = Enqueue Element(queue=w251, element=w250) -> (queue out=w249:refnum<queue>)  [unwired: 2 in, 2 out]
            }
          }
        }
      }
      frame "--move cursor" {
        n118 = in-place {
          in-place-border: w263 -> [_]
          n119 = in-place-cluster #11(w264) -> ("XY Graph"=w268:refnum<vi>, "set angle"=w266:dbl)
          n120 = Polar To Complex(1:w266, 2:1.3 ("r")) -> (0:w271:cdb)
          n121 = Complex To Re/Im(x + iy=w271) -> (x=w272:dbl, y=w273:dbl)
          n122 = call "replace cursor - plot ref - V2.vi"("Plot ref in"=w268, "new X"=w272, "new  Y"=w273, "cursor action"=cursor_action."write") -> ("Plot ref out"=w267:refnum<vi>)  [unwired: 12 in, 3 out]
          n123 = in-place-cluster #11("XY Graph"=w267, "set angle"=w266) -> (w265:T1)
        }
      }
      frame "check" {
        w276 = T3[] [enum."--move cursor"] items=["--update circle", "set step slider moves", "cursor moves", "current pos changed", "init", "void", "--draw current lie", "--draw set line", "--move current step slider", "--move set step slider", "--draw limit lines", "check", "--move set angle slider", "--move current angle slider", "set angle slider moves", "--move cursor", "set set step", "set current step"] ("action list IN")
        n124 = in-place {
          in-place-border: w277 -> [w287]
          n125 = in-place-cluster #12(w278) -> ("set pos slider"=w304:refnum<vi>, "current pos... slider"=w302:refnum<vi>, "set angle slider"=w301:refnum<vi>, "cur angle slider"=w300:refnum<vi>, "XY Graph"=w284:refnum<vi>)  [unwired: 1 out]
          n126 = call "slider-check.vi"("slider in"=w304, "slider action"=slider_action."check") -> ("slider out"=w291:refnum<vi>)  [unwired: 9 in, 4 out]
          n127 = call "slider-check.vi"("slider in"=w301, "slider action"=slider_action."check") -> ("slider out"=w293:refnum<vi>)  [unwired: 9 in, 4 out]
          n128 = call "slider-check.vi"("slider in"=w302, "slider action"=slider_action."copy range", "slider from"=w291) -> ("slider out"=w295:refnum<vi>)  [unwired: 8 in, 4 out]
          n129 = call "slider-check.vi"("slider in"=w300, "slider action"=slider_action."copy range", "slider from"=w293) -> ("slider out"=w298:refnum<vi>)  [unwired: 8 in, 4 out]
          n130 = call "slider-check.vi"("slider in"=w293, "slider action"=slider_action."set from slider", "slider from"=w291) -> ("slider out"=w292:refnum<vi>, "value OUT"=w288:dbl)  [unwired: 8 in, 3 out]
          n131 = call "slider-check.vi"("slider in"=w298, "slider action"=slider_action."set from slider", "slider from"=w295) -> ("slider out"=w297:refnum<vi>)  [unwired: 8 in, 4 out]
          n132 = expression code="(x/180.0)*pi" "degrees to radians"(w288) -> (w283:dbl)
          n133 = call "replace cursor - plot ref - V2.vi"("Plot ref in"=w284, "window IN"=w287, "cursor action"=cursor_action."zoom to X win") -> ("Plot ref out"=w289:refnum<vi>)  [unwired: 13 in, 3 out]
          n134 = call "replace cursor - plot ref - V2.vi"("Plot ref in"=w289, "window IN"=w287, "cursor action"=cursor_action."zoom to Y win") -> ("Plot ref out"=w286:refnum<vi>)  [unwired: 13 in, 3 out]
          n135 = in-place-cluster #12("set pos slider"=w291, "current pos... slider"=w295, "set angle slider"=w292, "cur angle slider"=w297, "XY Graph"=w286, "set angle"=w283) -> (w279:T1)
        }
        n136 = for {
          shift-right: [w280] -> w274
          shift-left: w275 -> [w282]
          tunnel: w276 -> [w281] mode=indexing
          tunnel: [w280] -> _ mode=indexing
          n137 = Enqueue Element(queue=w282, element=w281) -> (queue out=w280:refnum<queue>)  [unwired: 2 in, 2 out]
        }
      }
    }
    n138 = Get Queue Status(queue=w13) -> (queue out=w15:refnum<queue>, # elements in queue=w12:i32)  [unwired: 2 in, 6 out]
    n139 = Equal To 0?(x=w12) -> (x = 0?=w11:bool)
  }
  "stepper graphics internal state OUT" <- w1
  n140 = Release Queue(queue=w3) -> ()  [unwired: 2 in, 3 out]
